vi "Create DigiPattern File_SPI.vi"(6 "SPI_Mode":T1, 7 "Timeset between frms":u32=50, 8 "error in (no error)":errorcluster, 9 "Pattern Name":string, 10 "SPI FRM":refnum<class "SPI_Frame_Root.lvclass">[](array[class]), 11 "DigiPattern_Generator.lvclass":refnum<class "DigiPattern_Generator.lvclass">) -> (0 "error out":errorcluster, 3 "DigiPattern_Generator.lvclass out":refnum<class "DigiPattern_Generator.lvclass">)   [LabVIEW 2018, in "DigiPattern_Generator.lvclass"]
uses:
  DigiPattern_Generator.lvclass
  SPI/SPI Frame Root/SPI_Frame_Root.lvclass
  SPI/Config Read SPI/SPI_Mode.ctl
  DigiPattern_Generator.lvclass/DigiPattern_Generator.ctl
  SPI/Config Read SPI/Config_Read_SPI.lvclass
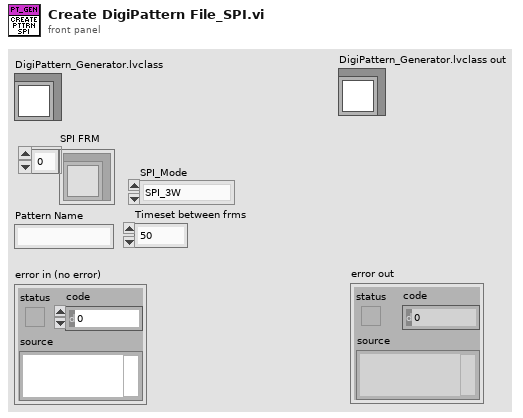
[diagram p1: front panel]
types:
  T1 = typedef "Config_Read_SPI.lvclass/SPI_Mode.ctl" = enum16{"SPI_3W", "SPI_4W"}
  T2 = enum32{"invalid app kind", "Development System", "Run Time System", "Student Edition", "Embedded LabVIEW", "Evaluation", "Custom"}
  T3 = enum16{"open", "replace", "create", "open or create", "replace or create", "replace or create with confirmation"}
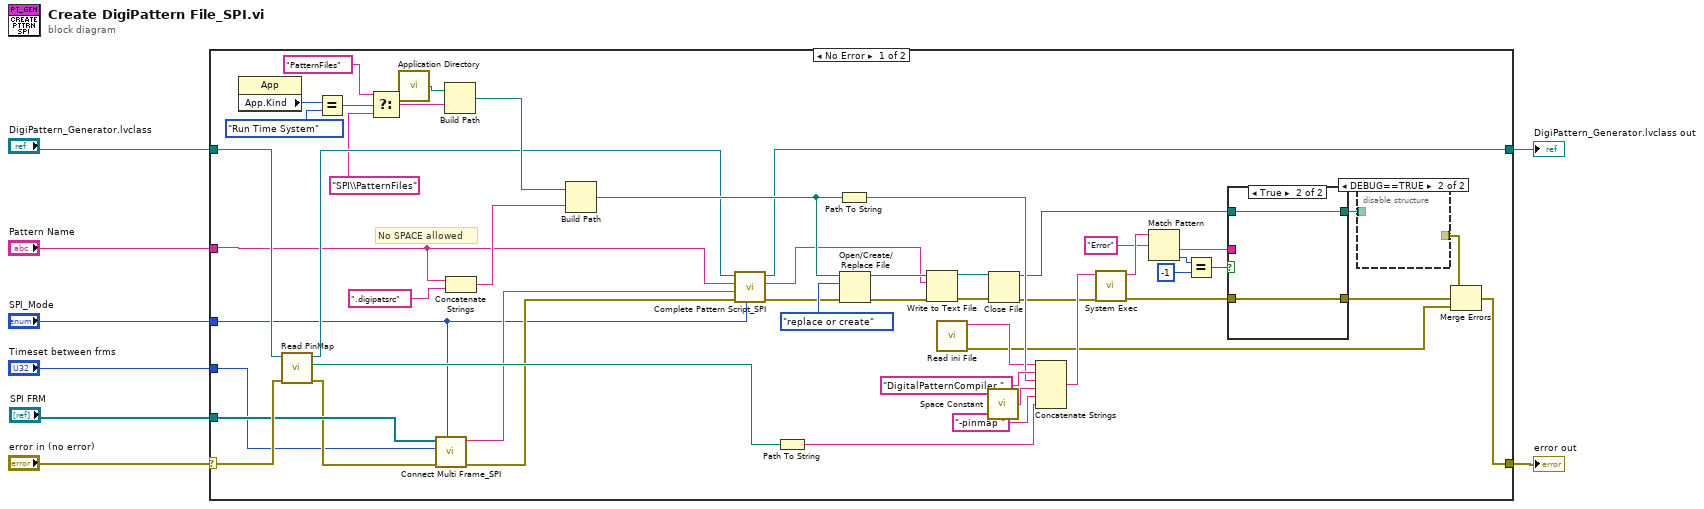
[diagram p0: block diagram]
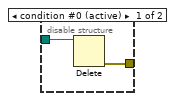
[diagram p2: hidden frame]
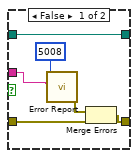
[diagram p3: hidden frame]
diagram:
  n1 = case shown="No Error" "error in (no error)" {
    selector: "error in (no error)" -> [w27 w71]
    tunnel: [w39 w71] -> w7
    tunnel: [w21 w70] -> w4
    tunnel: "DigiPattern_Generator.lvclass" -> [w28 w70]
    tunnel: "Pattern Name" -> [w20 _]
    tunnel: "SPI FRM" -> [w25 _]
    tunnel: "Timeset between frms" -> [w23 _]
    tunnel: "SPI_Mode" -> [w15 _]
    frame No Error {
      # "No SPACE allowed"
      n2 = property class="App"() -> ("App.Kind"=w14:T2)  [unwired: 2 in, 2 out]
      n3 = call "Read PinMap.vi"("error in (no error)"=w27, "BML_DigiPattern_Generator in"=w28) -> ("error out"=w24:errorcluster, "PinMap"=w26:path, "BML_DigiPattern_Generator out"=w22:refnum<class "DigiPattern_Generator.lvclass">)  [unwired: 7 in]
      n4 = Equal?(x=w14, y=T2."Run Time System") -> (x = y?=w12:bool)
      n5 = Select(t="PatternFiles" ("name or relative path"), s=w12, f="SPI\\PatternFiles" ("name or relative path")) -> (s? t:f=w9:string)
      n6 = call <vilib>:"Application Directory.vi"() -> ("Application Directory"=w35:path)
      n7 = call "Connect Multi Frame_SPI.vi"("SPI_Mode"=w15, "error in (no error)"=w24, "Timeset between frms"=w23, "SPI Frame Array"=w25) -> ("error out"=w18:errorcluster, "Connected Frame Contents"=w19:string)  [unwired: 6 in]
      n8 = Build Path(base path=w35, name or relative path=w9) -> (appended path=w34:path)
      n9 = Concatenate Strings(w20, ".digipatsrc" ("string")) -> (w58:string)
      n10 = Build Path(base path=w34, name or relative path=w58) -> (appended path=w53:path)
      n11 = call "Complete Pattern Script_SPI.vi"("SPI_Mode"=w15, "error in (no error)"=w18, "Pattern Contents"=w19, "Pattern Name"=w20, "DigiPattern_Generator.lvclass"=w22) -> ("error out"=w17:errorcluster, "All Pattern Script out"=w16:string, "DigiPattern_Generator.lvclass out"=w21:refnum<class "DigiPattern_Generator.lvclass">)  [unwired: 4 in]
      n12 = Path To String(path=w26) -> (string=w49:string)
      n13 = Path To String(path=w53) -> (string=w52:string)
      n14 = Open/Create/Replace File(file path (use dialog)=w53, error in=w17, operation (0:open)=T3."replace or create") -> (refnum out=w56:refnum<file>, error out=w55:errorcluster)  [unwired: 3 in, 1 out]
      n15 = Write to Text File(file (use dialog)=w56, text=w16, error in=w55) -> (refnum out=w38:refnum<file>, error out=w37:errorcluster)  [unwired: 1 in, 1 out]
      n16 = call "Read ini File.vi"() -> ("error out"=w29:errorcluster, "value"=w30:string)  [unwired: 10 in]
      n17 = call <vilib>:"Space Constant.vi"() -> ("String"=w51:string)
      n18 = Close File(refnum=w38, error in=w37) -> (path=w32:path, error out=w36:errorcluster)
      n19 = Concatenate Strings(w30, "DigitalPatternCompiler " ("string"), w52, w51, "-pinmap " ("string"), w49) -> (w48:string)
      n20 = call <vilib>:"System Exec.vi"("error in (no error)"=w36, "command line"=w48) -> ("error out"=w41:errorcluster, "standard output"=w47:string)  [unwired: 6 in, 2 out]
      n21 = Match Pattern(string=w47, regular expression="Error") -> (after substring=w42:string, offset past match=w45:i32)  [unwired: 1 in, 2 out]
      n22 = Equal?(x=w45, y=-1) -> (x = y?=w43:bool)
      n23 = case shown="True" w43 {
        tunnel: w42 -> [w63 _]
        tunnel: w41 -> [w67 w69]
        tunnel: [w66 w69] -> w40
        tunnel: w32 -> [w65 w68]
        tunnel: [w65 w68] -> w31
        frame False {
          n24 = call "Error Report.vi"("Additional info"=w63, "Error Code"=i16 5008) -> ("error out"=w62:errorcluster)  [unwired: 9 in]
          n25 = Merge Errors(w62, w67) -> (w66:errorcluster)
        }
        frame True {
        }
      }
      n26 = disable-structure shown="DEBUG==TRUE" {
        disable-tunnel: [w61 _] -> w33
        disable-tunnel: w31 -> [w60 _]
        frame condition #0 (active) {
          n27 = Delete(path (use dialog)=w60) -> (error out=w61:errorcluster)  [unwired: 4 in, 2 out]
        }
        frame condition #1 {
        }
      }
      n28 = Merge Errors(w33, w40, w29) -> (w39:errorcluster)
    }
    frame Error {
    }
  }
  "error out" <- w7
  "DigiPattern_Generator.lvclass out" <- w4
